vi "Patch data preview-Sync scrollbars.vi"(7 "Min cursor moved":bool, 8 "error in (no error)":errorcluster, 11 "Scrollbar value":i32) -> (0 "error out":errorcluster)   [LabVIEW 2017]
uses:
  Globals/gl_Funct viewer (patches) globals.vi
panel:
  out "Extractor slider":cluster{"Min cursor":i32, "Max cursor":i32}
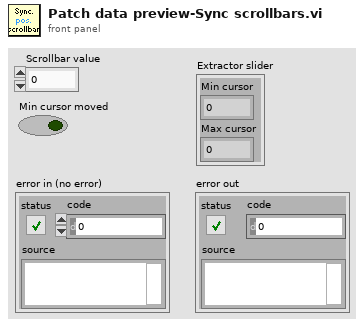
[diagram p1: front panel]
types:
  T1 = typedef "Patch viewer refs.ctl" = cluster{"This VI":refnum<vi>, "AVI Mode ind":refnum<vi>, "Play":refnum<vi>, "Stop":refnum<vi>, "Back":refnum<vi>, "Scrollbar":refnum<vi>, "Video length info":refnum<vi>, "Expected speed values":refnum<vi>, "Intensity":refnum<vi>, "Path":refnum<vi>, "Selection sliders":refnum<vi>, "Speed Graph ref":refnum<vi>, "Frame rate set (fps)":refnum<vi>, "Number of rows to generate":refnum<vi>, "Channel to load":refnum<vi>, "Peak value in dataset":refnum<vi>}
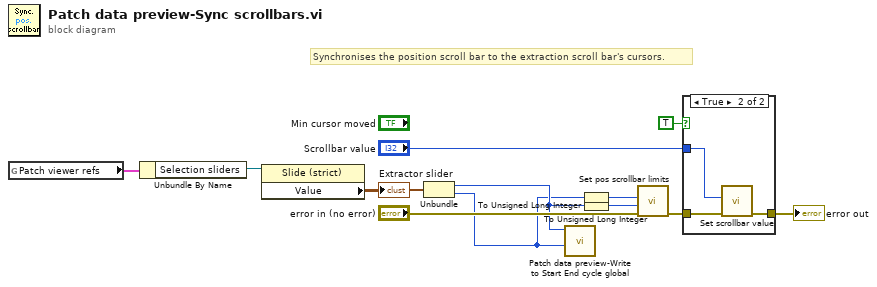
[diagram p0: block diagram]
diagram:
  # "Synchronises the position scroll bar to the extraction scroll bar's cursors."
  n1 = global read "gl_Funct viewer (patches) globals.vi" "Patch viewer refs"() -> (w1:T1)
  n2 = Unbundle By Name(w1) -> ("Selection sliders"=w5:refnum<vi>)
  n3 = property class="Slide (strict)"(reference=w5) -> ("Value"=w4:cluster{i32, i32})  [unwired: 1 in, 2 out]
  "Extractor slider" <- w4
  n4 = Unbundle(w4) -> (w3:i32, w2:i32)
  n5 = call "Patch data preview-Write to Start End cycle global.vi"("Max cursor / End cycle"=w2, "Min cursor / Start cycle"=w3) -> ()  [unwired: 10 in]
  n6 = To Unsigned Long Integer(number=w2) -> (unsigned 32bit integer=w7:u32)
  n7 = To Unsigned Long Integer(number=w3) -> (unsigned 32bit integer=w6:u32)
  n8 = call "Set pos scrollbar limits.vi"("error in (no error)"="error in (no error)", "Min frame (unity-based)"=w6, "Max frame (unity-based)"=w7) -> ("error out"=w11:errorcluster)  [unwired: 8 in]
  n9 = case shown="True" TRUE {
    tunnel: "Scrollbar value" -> [_ w16]
    tunnel: w11 -> [w13 w15]
    tunnel: [w13 w14] -> w10
    frame False {
    }
    frame True {
      n10 = call "Set scrollbar value.vi"("error in (no error)"=w15, "Scrollbar value"=w16) -> ("error out"=w14:errorcluster)  [unwired: 9 in]
    }
  }
  "error out" <- w10
